vi "Host3.vi"() -> ()   [LabVIEW 2025]
uses:
  <vilib>/numeric/Random Number (Range) U64.vi
  <vilib>/Analysis/baseanly.llb/Real Dot Product.vi
  <vilib>/Analysis/baseanly.llb/Real A x B.vi
  <vilib>/numeric/sub_Random U32.vi
  <vilib>/Analysis/Matrix/Numeric/Conversions/Matrix To Array - RM.vi
  <vilib>/FPGAPlugInAG/cRIO-9033/niLvFpga_Open_cRIO-9033.vi
  <vilib>/rvi/interface/common/dynamic/niFpgaDynamicAddResources.vi
  <vilib>/FPGAPlugInAG/Dynamic/niLvFpga_Reset_Dynamic.vi
  <vilib>/Utility/error.llb/Error Cluster From Error Code.vi
  <vilib>/rvi/errors/niLvFpgaAdjustHostInterfaceError.vi
  <vilib>/FPGAPlugInAG/Dynamic/niLvFpga_Run_Dynamic.vi
  <vilib>/FPGAPlugInAG/Dynamic/niLvFpga_Close_Dynamic.vi
  <vilib>/rvi/interface/nirviOpenFPGA/nirviOpenFPGA.xnode
  FPGA Bitfiles/dotplot9033_FPGATarget_Target3_Uh+3i-uoQCI.lvbitx
  Target3.vi
  <vilib>/rvi/interface/nirviMethod/nirviMethod.xnode
  <vilib>/rvi/interface/nirviReadWriteControl/nirviReadWriteControl.xnode
  <vilib>/rvi/interface/nirviCloseFPGA/nirviCloseFPGA.xnode
  <vilib>/rvi/errors/niLvFpgaMergeErrorWithErrorCode.vi
  <vilib>/Analysis/NI_AALBase.lvlib
  <vilib>/Analysis/Matrix/NI_Matrix.lvlib
  <vilib>/FPGAPlugInAG/Dynamic/niLvFpga_WriteFifo_Dynamic.vi
  <vilib>/FPGAPlugInAG/Dynamic/niLvFpga_ReadFifo_Dynamic.vi
  NiFpgaLv.dll
  <vilib>/rvi/interface/Simulation/niFpgaSimulationCallBeginRW.vi
panel:
  out "And 2":bool[](array[boolean])
  out "And 1":bool[](array[boolean])
  out "ready for a":bool[](array[boolean])
  out "ready for b":bool[](array[boolean])
  out "element 2":fxp<+/-,32,16>
  out "element":fxp<+/-,32,16>
  out "cr":fxp<+/-,32,16>[](array[numeric])
  out "Numeric 2":i32
  out "Array 3":fxp<+/-,32,16>[](array[numeric])
  out "Ready for Input":bool
  out "output valid":bool
  out "Numeric":i32
  out "Elements Remaining":u32
  out "appended array 2":fxp<+/-,32,16>[](array[numeric])
  out "appended array":fxp<+/-,32,16>[](array[numeric])
  out "Array B":fxp<+/-,32,16>[](array[numeric])
  out "Array A":fxp<+/-,32,16>[](array[numeric])
  out "FIFO C Output":fxp<+/-,32,16>[](array[numeric])
  out "FIFO A Input":fxp<+/-,32,16>[](array[numeric])
  out "FIFO B Input":fxp<+/-,32,16>[](array[numeric])
  out "X * Y":fxp<+/-,64,32>
  out "elements in B":i32
  out "elements in A":i32
  out "sum of error":dbl
  out "C - FPGA code":fxp<+/-,32,16>[][](array[numeric])
  out "elements in C":i32
  out "C - Real":dbl[][](array[numeric])
  out "B":fxp<+/-,32,16>[][](array[numeric])
  out "A":fxp<+/-,32,16>[][](array[numeric])
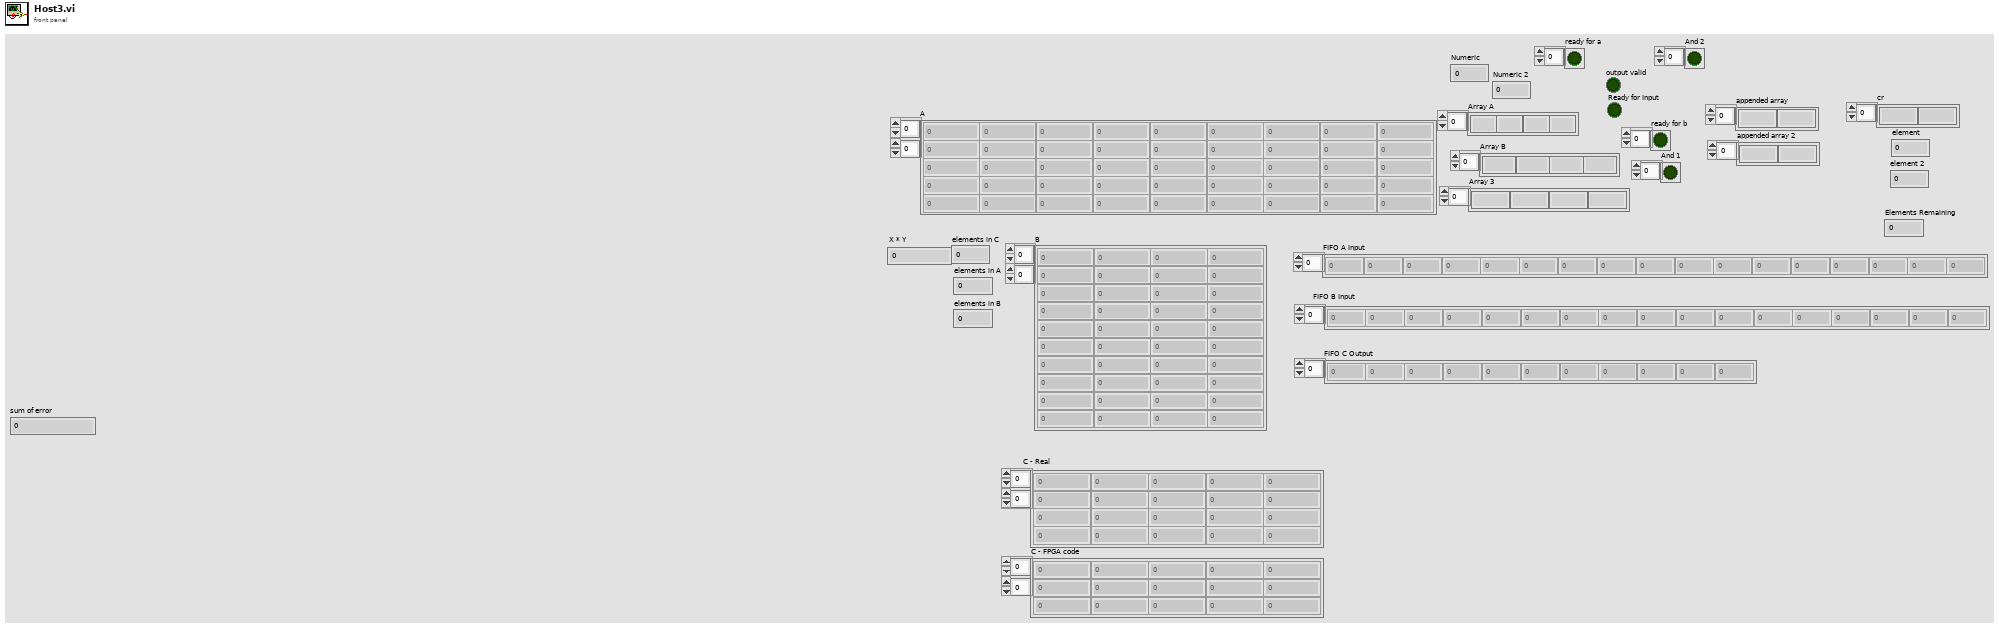
[diagram p1: front panel]
types:
  T1 = typedef "NI_Matrix.lvlib/RealMatrix.ctl" = dbl[][]
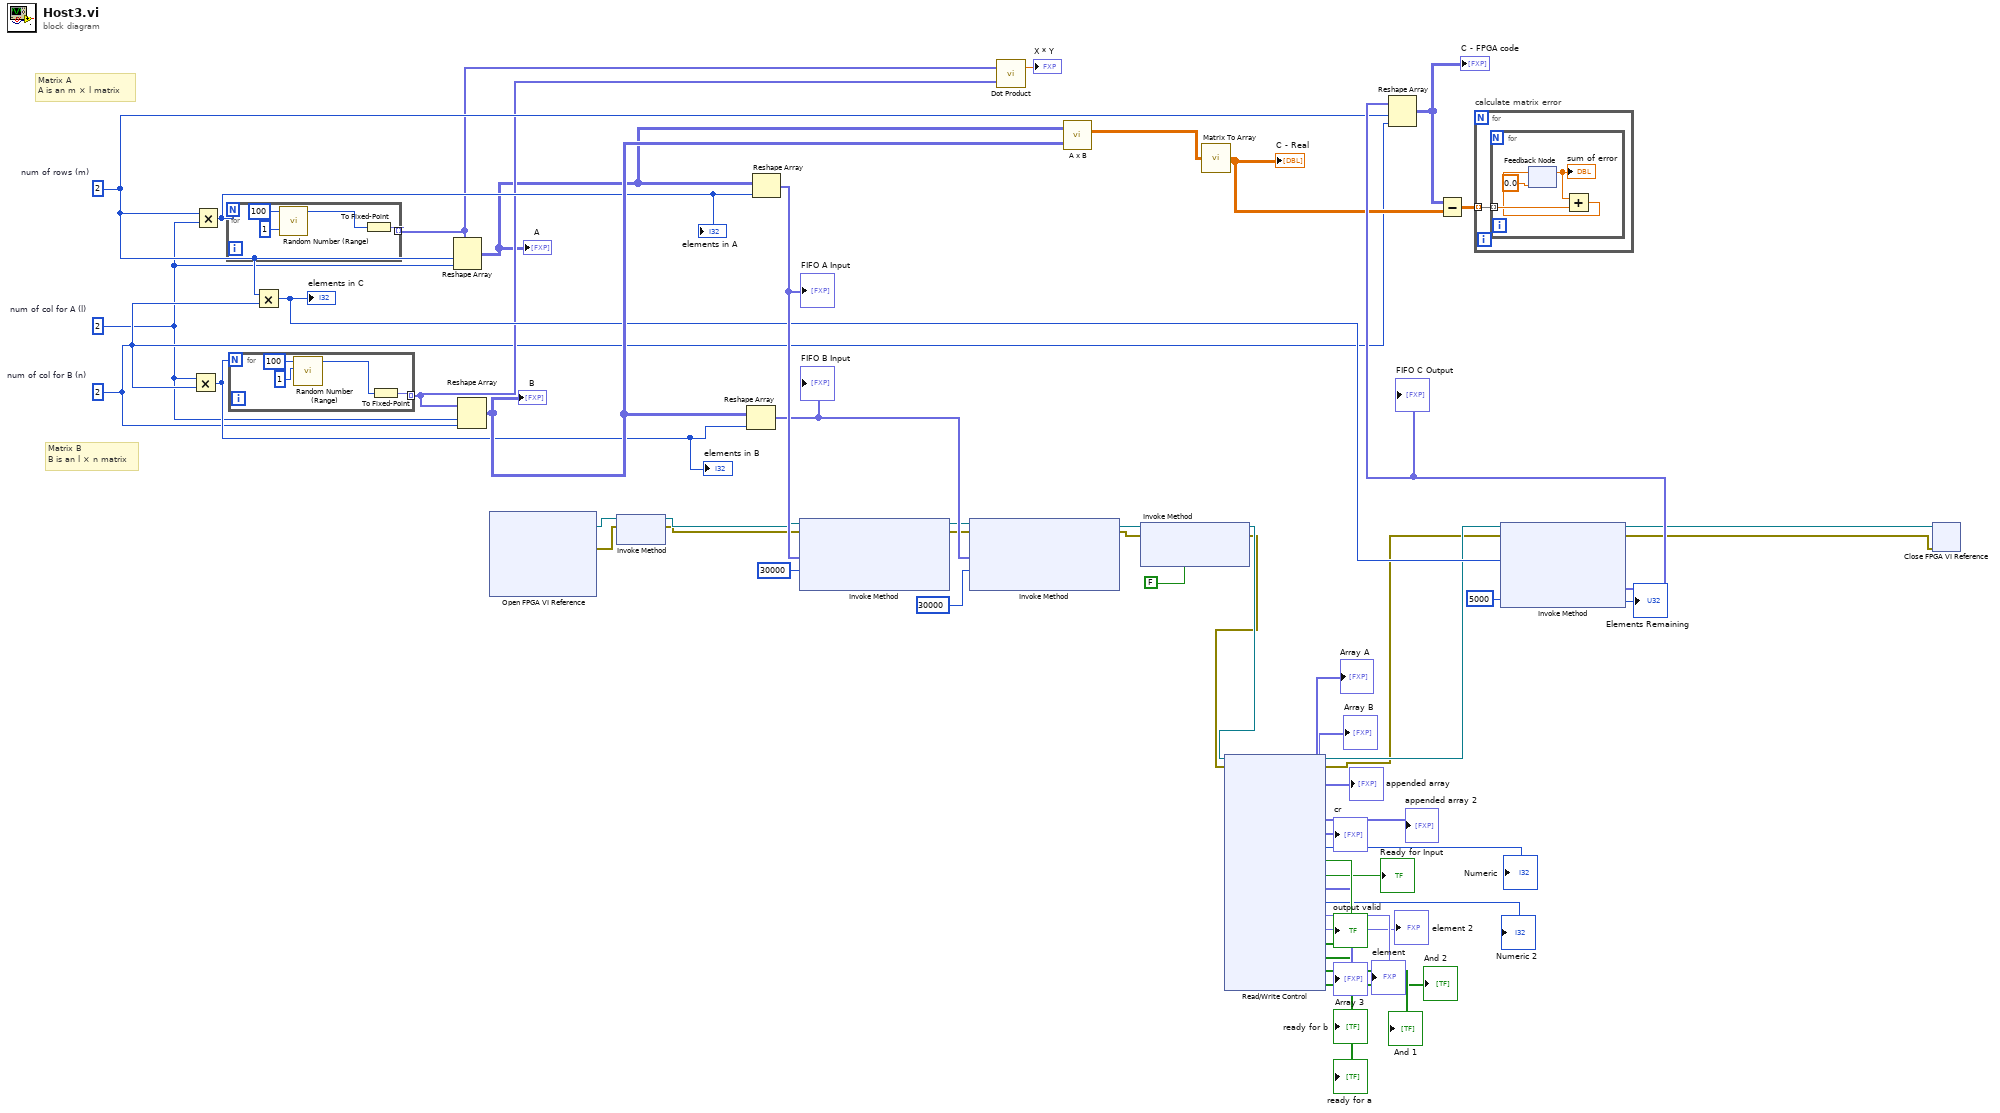
[diagram p0: block diagram]
diagram:
  w38 = 2  # num of col for B (n)
  w37 = 2  # num of col for A (l)
  w46 = 2  # num of rows (m)
  # "Matrix B\nB is an l × n matrix"
  # "Matrix A\nA is an m × l matrix"
  n1 = Multiply(x=w37, y=w38) -> (x*y=w43:i32)
  "elements in B" <- w43
  n2 = Multiply(x=w46, y=w37) -> (x*y=w51:i32)
  "elements in A" <- w51
  n3 = for {
    N: w51 -> [_]
    tunnel: [w57] -> w42 mode=indexing
    n4 = call-poly <vilib>:"Random Number (Range).vi"("lower bound (0)"=u64 1, "upper bound (100)"=u64 100) -> ("number"=w56:u64)  [unwired: 9 in]
    n5 = To Fixed-Point(number=w56) -> (fixed-point=w57:fxp<+,64,64>)  [unwired: 1 in]
  }
  n6 = for {
    N: w43 -> [_]
    tunnel: [w61] -> w41 mode=indexing
    n7 = call-poly <vilib>:"Random Number (Range).vi"("lower bound (0)"=u64 1, "upper bound (100)"=u64 100) -> ("number"=w58:u64)  [unwired: 9 in]
    n8 = To Fixed-Point(number=w58) -> (fixed-point=w61:fxp<+,64,64>)  [unwired: 1 in]
  }
  n9 = Multiply(x=w46, y=w38) -> (x*y=w44:i32)
  "elements in C" <- w44
  n10 = Reshape Array(w42, w46, w37) -> (w39:fxp<+,64,64>[][])
  "A" <- w39
  n11 = Reshape Array(w41, w37, w38) -> (w53:fxp<+,64,64>[][])
  "B" <- w53
  n12 = xnode "Open FPGA VI Reference"() -> ("FPGA VI Reference Out"=w35:refnum<k20>, "error out"=w32:errorcluster)  [unwired: 2 in]
  n13 = xnode "Invoke Method"("FPGA VI Reference In"=w35, "error in"=w32) -> ("FPGA VI Reference Out"=w34:refnum<k20>, "error out"=w33:errorcluster)
  n14 = Reshape Array(w53, w43) -> (w36:fxp<+,64,64>[])
  "FIFO B Input" <- w36
  n15 = Reshape Array(w39, w51) -> (w50:fxp<+,64,64>[])
  "FIFO A Input" <- w50
  n16 = xnode "Invoke Method"("FPGA VI Reference In"=w34, "error in"=w33, "Data"=w50, "Timeout (ms)"=30000) -> ("FPGA VI Reference Out"=w27:refnum<k20>, "error out"=w26:errorcluster)  [unwired: 1 out]
  n17 = xnode "Invoke Method"("FPGA VI Reference In"=w27, "error in"=w26, "Data"=w36, "Timeout (ms)"=30000) -> ("FPGA VI Reference Out"=w30:refnum<k20>, "error out"=w29:errorcluster)  [unwired: 1 out]
  n18 = call-poly <vilib>:"Dot Product.vi"("Y Vector"=w41, "X Vector"=w42) -> ("X * Y"=→"X * Y":dbl)  [unwired: 1 out]
  n19 = call-poly <vilib>:"A x B.vi"("B"=w53, "A"=w39) -> ("A x B"=w52:T1)  [unwired: 1 out]
  n20 = xnode "Invoke Method"("FPGA VI Reference In"=w30, "error in"=w29, "Wait Until Done (F)"=FALSE) -> ("FPGA VI Reference Out"=w17:refnum<k20>, "error out"=w16:errorcluster)
  n21 = call-poly <vilib>:"Matrix To Array.vi"("Real Matrix"=w52) -> ("Real 2D Array"=w45:dbl[][])
  "C - Real" <- w45
  n22 = xnode "Read/Write Control"("FPGA VI Reference In"=w17, "error in"=w16) -> ("FPGA VI Reference Out"=w19:refnum<k20>, "error out"=w18:errorcluster, "Array 5"=→"Array A":fxp<+/-,32,16>[], "Array 4"=→"Array B":fxp<+/-,32,16>[], "appended array"=→"appended array":fxp<+/-,32,16>[], "appended array 2"=→"appended array 2":fxp<+/-,32,16>[], "cr"=→"cr":fxp<+/-,32,16>[], "Numeric"=→"Numeric":i32, "output valid"=→"output valid":bool, "Ready for Input"=→"Ready for Input":bool, "Array 3"=→"Array 3":fxp<+/-,32,16>[], "Numeric 2"=→"Numeric 2":i32, "element"=→"element":fxp<+/-,32,16>, "element 2"=→"element 2":fxp<+/-,32,16>, "ready for b"=→"ready for b":bool[], "ready for a"=→"ready for a":bool[], "And 1"=→"And 1":bool[], "And 2"=→"And 2":bool[])
  n23 = xnode "Invoke Method"("FPGA VI Reference In"=w19, "error in"=w18, "Number of Elements"=w44, "Timeout (ms)"=5000) -> ("FPGA VI Reference Out"=w15:refnum<k20>, "error out"=w14:errorcluster, "Data"=w47:fxp<+/-,32,16>[], "Elements Remaining"=→"Elements Remaining":u32)
  "FIFO C Output" <- w47
  n24 = Reshape Array(w47, w46, w38) -> (w49:fxp<+/-,32,16>[][])
  "C - FPGA code" <- w49
  n25 = Subtract(x=w49, y=w45) -> (x-y=w48:dbl[][])
  n26 = for "calculate matrix error" {
    tunnel: w48 -> [w62] mode=indexing
    n27 = for {
      tunnel: w62 -> [w66] mode=indexing
      n28 = feedback #1(0.0) -> (w64:dbl)
      "sum of error" <- w64
      n29 = Add(x=w64, y=w66) -> (x+y=w65:dbl)
      n30 = feedback-in #1(w65) -> ()
    }
  }
  n31 = xnode "Close FPGA VI Reference"("FPGA VI Reference In"=w15, "error in"=w14) -> ()  [unwired: 1 out]
